vi "Arrival_time_weighting.vi"(1 "Arrival times":dbl[](array[numeric]) format="%.2f") -> (0 "Weighting":dbl[](array[numeric]) format="%.2f")   [LabVIEW 2010]
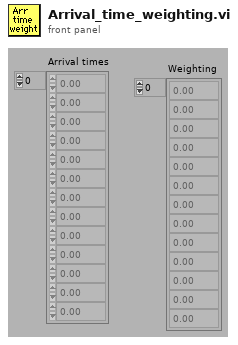
[diagram p1: front panel]
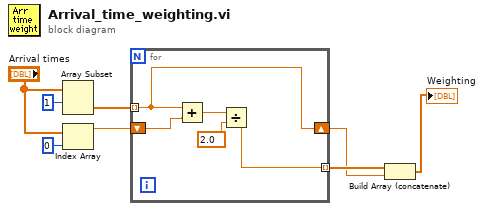
[diagram p0: block diagram]
diagram:
  n1 = Array Subset(array="Arrival times", index=1) -> (w4:dbl[])  [unwired: 1 in]
  n2 = Index Array(array="Arrival times", index=0) -> (element=w7:dbl)
  n3 = for {
    shift-right: [w9] -> w1
    shift-left: w7 -> [w13]
    tunnel: w4 -> [w9] mode=indexing
    tunnel: [w10] -> w3 mode=indexing
    n4 = Add(x=w9, y=w13) -> (x+y=w12:dbl)
    n5 = Divide(x=w12, y=2.0) -> (x/y=w10:dbl)
  }
  n6 = Build Array (concatenate)(w3, w1) -> (→"Weighting":dbl[])
